vi "GPS_file_Init.vi"(11 "file path (dialog if empty)":path) -> (2 "Header":string[](array[string]), 3 "Data":string[][](array[string]))   [LabVIEW 2019]
uses:
  <vilib>/Utility/file.llb/Write Delimited Spreadsheet (string).vi
  <vilib>/Utility/file.llb/Read Delimited Spreadsheet (string).vi
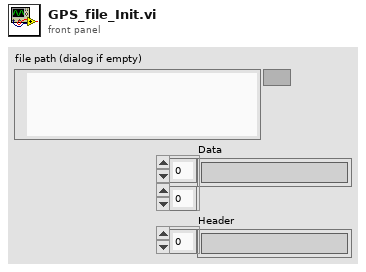
[diagram p1: front panel]
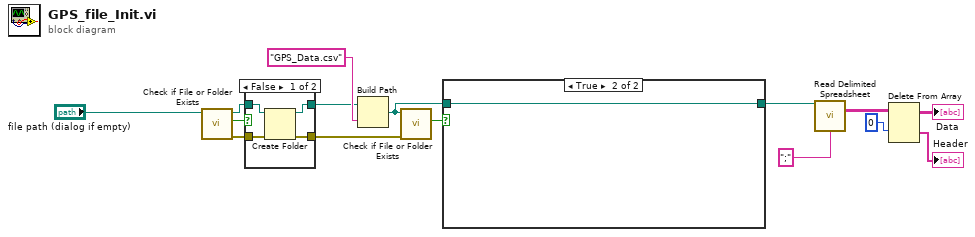
[diagram p0: block diagram]
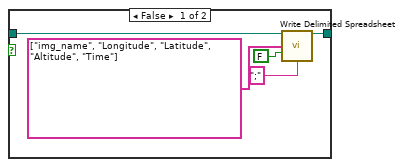
[diagram p3: hidden frame]
diagram:
  n1 = call <vilib>:"Check if File or Folder Exists.vi"("path"="file path (dialog if empty)") -> ("error out"=w9:errorcluster, "file or folder exists?"=w11:bool, "dup path"=w10:path)  [unwired: 8 in]
  n2 = case shown="False" w11 {
    tunnel: [w18 w21] -> w7
    tunnel: w10 -> [w19 w21]
    tunnel: w9 -> [w17 w20]
    tunnel: [w16 w20] -> w8
    frame False {
      n3 = Create Folder(path (use dialog)=w19, error in=w17) -> (created path=w18:path, error out=w16:errorcluster)  [unwired: 1 in, 1 out]
    }
    frame True {
    }
  }
  n4 = Build Path(base path=w7, name or relative path="GPS_Data.csv") -> (appended path=w13:path)
  n5 = call <vilib>:"Check if File or Folder Exists.vi"("error in (no error)"=w8, "path"=w13) -> ("file or folder exists?"=w14:bool)  [unwired: 7 in, 2 out]
  n6 = case shown="True" w14 {
    tunnel: w13 -> [w26 w27]
    tunnel: [w22 w27] -> w5
    frame False {
      n7 = call-poly <vilib>:"Write Delimited Spreadsheet.vi"("file path (dialog if empty)"=w26, "1D data"=string[] ["img_name", "Longitude", "Latitude", "Altitude", "Time"], "append to file? (new file:F)"=FALSE, "delimiter (\\t)"=";" ("delimiter (\\t)")) -> ("new file path (Not A Path if cancelled)"=w22:path)  [unwired: 10 in, 1 out]
    }
    frame True {
    }
  }
  n8 = call-poly <vilib>:"Read Delimited Spreadsheet.vi"("file path (dialog if empty)"=w5, "delimiter (\\t)"=";" ("delimiter (\\t)")) -> ("all rows"=w4:string[][])  [unwired: 8 in, 5 out]
  n9 = Delete From Array(array=w4, index (row)=0) -> (deleted portion=→"Header":string[], array with subset deleted=→"Data":string[][])  [unwired: 2 in]
